vi "load_single_image.vi"(11 "Path":path) -> (0 "error out":errorcluster, 3 "Refnum out":T1)   [LabVIEW 2017]
uses:
  <vilib>/vision/Image Controls.llb/IMAQ Image.ctl
panel:
  in  "error in":errorcluster
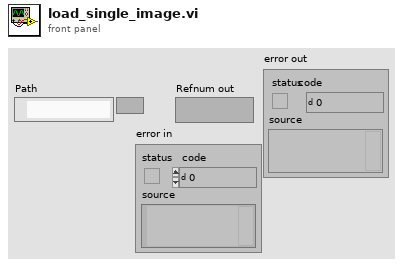
[diagram p1: front panel]
types:
  T1 = typedef "IMAQ Image.ctl" = refnum<image>
  T2 = typedef "Image Type" = u32
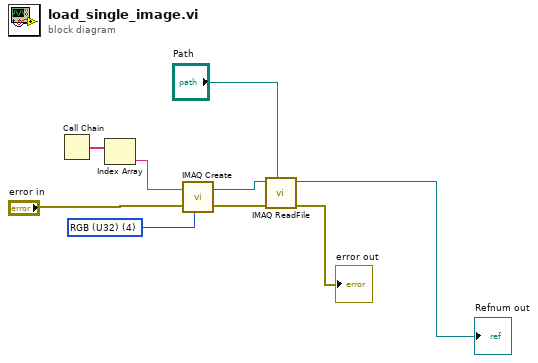
[diagram p0: block diagram]
diagram:
  w6 = T2 4 items=["Grayscale (U8)", "Grayscale (I16)", "Grayscale (SGL)", "Complex (CSG)", "RGB (U32)", "HSL (U32)", "RGB (U64)", "Grayscale (U16)"] ("Image Type")
  n1 = Call Chain() -> (call chain=w4:string[])
  n2 = Index Array "Index Array"(array=w4) -> (element=w5:string)  [unwired: 1 in]
  n3 = call "IMAQ Create"("Image Name"=w5, "Image Type"=w6, "error in (no error)"="error in") -> ("New Image"=w7:T1, "error out"=w3:errorcluster)  [unwired: 1 in, 1 out]
  n4 = call "IMAQ ReadFile"("File Path"="Path", "error in (no error)"=w3, "Image"=w7) -> ("error out"=→"error out":errorcluster, "Image Out"=→"Refnum out":T1)  [unwired: 2 in, 5 out]
